vi "_test Dialog.vi"() -> ()   [LabVIEW 2012]
uses:
  Dialog/Dialog/Dialog/Dialog.lvclass
panel:
  in  "Timeout (-1)":i32=2000
  in  "Message":string="hdsfghjdfhsdhdhhdfghdhdsfhdh"
  in  "Dialog Title":string="hjdfjhdfjhd"
  out "error out":errorcluster
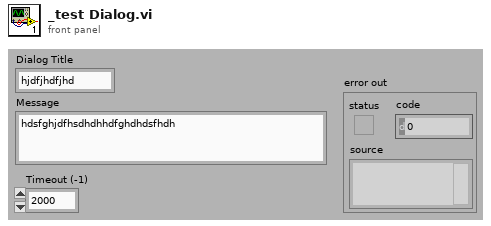
[diagram p1: front panel]
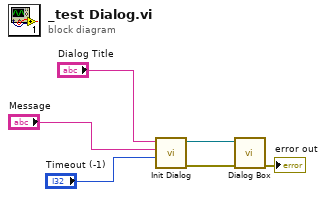
[diagram p0: block diagram]
diagram:
  n1 = call "Init Dialog.vi"("Timeout (-1)"="Timeout (-1)", "Message"="Message", "Dialog Title"="Dialog Title") -> ("error out"=w2:errorcluster, "Dialog out"=w6:refnum<class "Dialog.lvclass">)  [unwired: 3 in, 4 out]
  n2 = call-dynamic "Dialog Box.vi"("error in (no error)"=w2, "Dialog in"=w6) -> ("error out"=→"error out":errorcluster)  [unwired: 9 out]
